vi "Test Comm.vi"() -> ()   [LabVIEW 2021]
uses:
  CIFChannels/Typedef/Direction.ctl
  ChannelCommon/typedef/FIFO Config.ctl
  ChannelCommon/typedef/Datatype Waveform.ctl
  ChannelCommon/typedef/TimeStamps.ctl
  CIF_NIChn_FIFO_DAQ.lvclass
  <vilib>/CIF Foundation/CIF Utilities/DataTypes/Flatten U64.vi
  ChannelCommon/ChannelCommon.lvlib
  CIFChannels/CIFChannels.lvclass
panel:
  out "status":string
  out "pass":bool
  out "error out":errorcluster
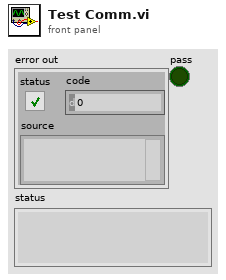
[diagram p1: front panel]
types:
  T1 = typedef "CIFChannels.lvclass/Direction.ctl" = enum16{"Publisher", "Subscriber"}
  T2 = typedef "ChannelCommon.lvlib/TimeStamps.ctl" = cluster{"ClockID":u8, "T0":i64, "T_Out":i64}
  T3 = typedef "ChannelCommon.lvlib/FIFO Config.ctl" = cluster{"Max Bytes/Msg":u64, "Max Msg/FIFO":u64, "Flags":u64}
  T4 = typedef "ChannelCommon.lvlib/Datatype Waveform.ctl" = cluster{"measurement":dbl[], "dT":dbl, "Timestamp":i64, "Read Lock":bool}
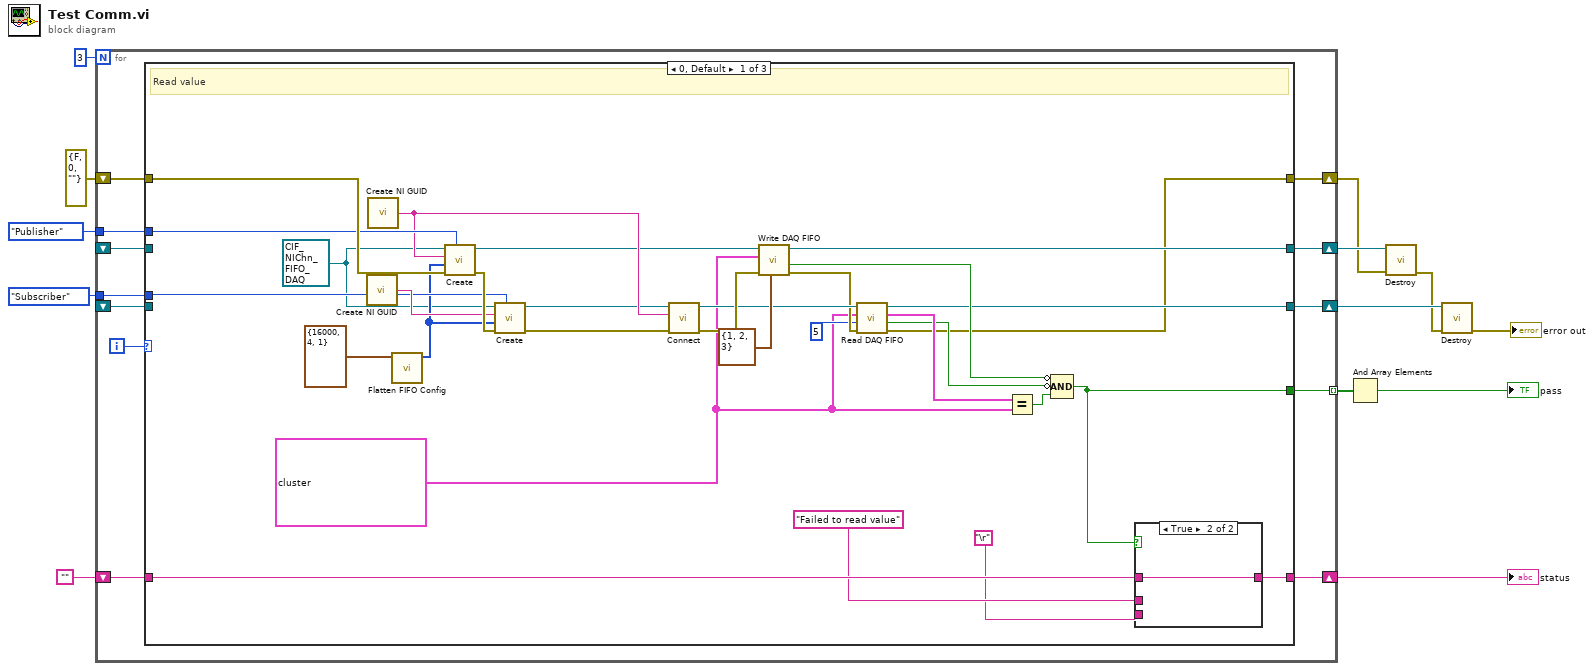
[diagram p0: block diagram]
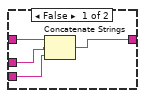
[diagram p2: hidden frame]
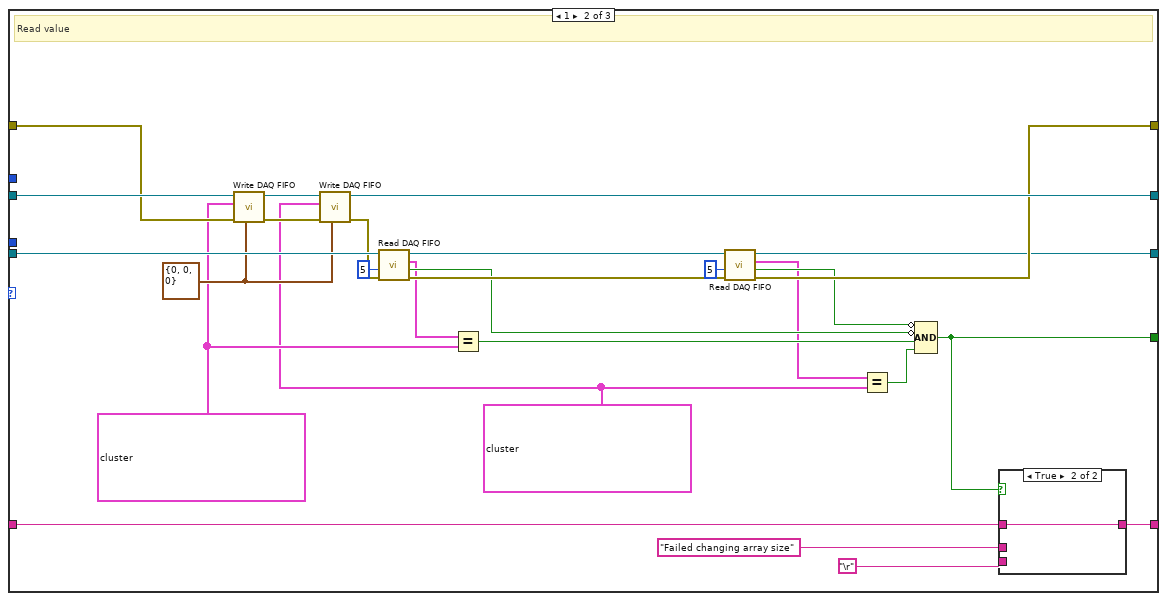
[diagram p3: hidden frame]
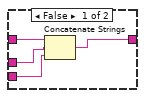
[diagram p4: hidden frame]
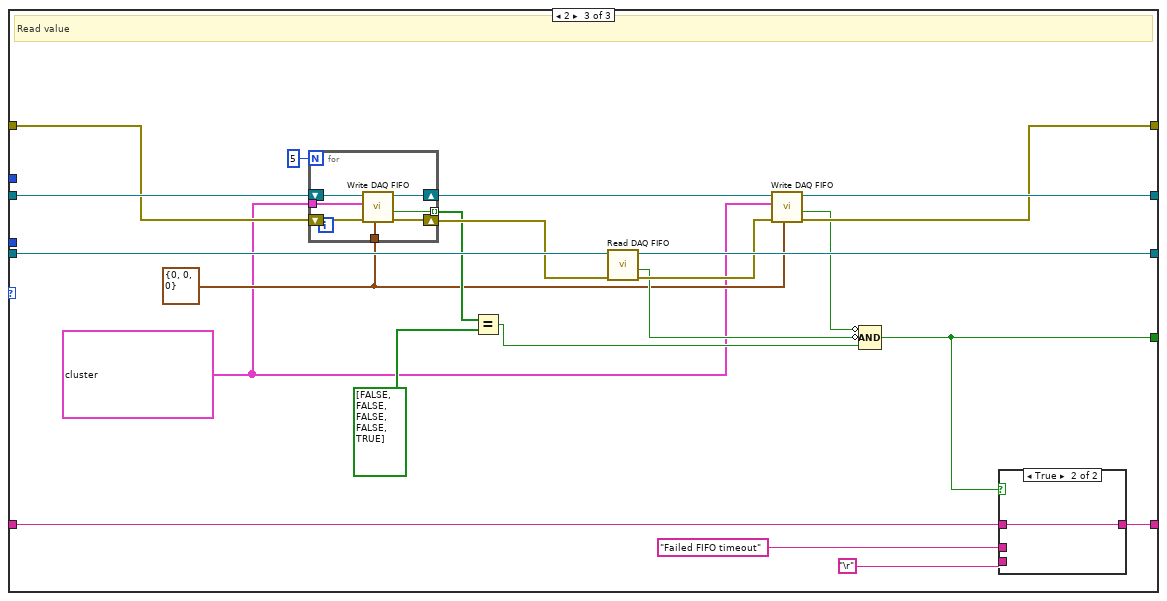
[diagram p5: hidden frame]
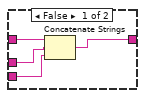
[diagram p6: hidden frame]
diagram:
  n1 = for {
    N: 3 -> [_]
    tunnel: [w25] -> w13 mode=indexing
    shift-right: [w14] -> w3
    shift-left: errorcluster {"status"=FALSE, "code"=0, "source"=""} ("error out") -> [w24]
    shift-right: [w21] -> w9
    shift-left: "" -> [w22]
    tunnel: Direction."Subscriber" ("Direction") -> [w20]
    tunnel: Direction."Publisher" ("Direction") -> [w19]
    shift-right: [w18] -> w5
    shift-left: _ -> [w16]
    shift-right: [w17] -> w4
    shift-left: _ -> [w15]
    i -> [w23]
    n2 = case shown="0, Default" w23 {
      tunnel: [w50 w83 w95] -> w25
      tunnel: w24 -> [w48 w79 w109]
      tunnel: [w28 w72 w101] -> w14
      tunnel: w22 -> [w55 w87 w114]
      tunnel: [w54 w86 w113] -> w21
      tunnel: w20 -> [w46 _ _]
      tunnel: w19 -> [w45 _ _]
      tunnel: [w30 w69 w106] -> w18
      tunnel: [w36 w76 w104] -> w17
      tunnel: w15 -> [_ w80 w110]
      tunnel: w16 -> [_ w75 w107]
      frame 0, Default {
        w26 = refnum<class "CIF_NIChn_FIFO_DAQ.lvclass"> refnum ("CIF_NIChn_FIFO_DAQ.lvclass")
        w27 = T4[] [{"measurement"=array[986 elements], "dT"=43.0, "Timestamp"=2, "Read Lock"=FALSE}, {"measurement"=array[1001 elements], "dT"=34.0, "Timestamp"=1, "Read Lock"=FALSE}] ("DAQ In")
        # "Read value"
        n3 = call <vilib>:"Create NI GUID.vi"() -> ("NI GUID"=w47:string)
        n4 = call <vilib>:"Create NI GUID.vi"() -> ("NI GUID"=w43:string)
        n5 = call "Flatten FIFO Config.vi"("FIFO Config in"=T3 {"Max Bytes/Msg"=16000, "Max Msg/FIFO"=4, "Flags"=1}) -> ("Flattened FIFO Config"=w40:u8[])  [unwired: 10 in]
        n6 = call-dynamic "Create.vi"("Direction"=w45, "error in (no error)"=w48, "Custom Config Data"=w40, "Name"=w43, "CIFFIFO in"=w26) -> ("error out"=w49:errorcluster, "CIFFIFO out"=w39:refnum<class "CIF_NIChn_FIFO_DAQ.lvclass">)  [unwired: 5 in]
        n7 = call-dynamic "Create.vi"("Direction"=w46, "error in (no error)"=w49, "Custom Config Data"=w40, "Name"=w47, "CIFFIFO in"=w26) -> ("error out"=w42:errorcluster, "CIFFIFO out"=w41:refnum<class "CIF_NIChn_FIFO_DAQ.lvclass">)  [unwired: 5 in]
        n8 = call-dynamic "Connect.vi"("error in (no error)"=w42, "Connection Name"=w43, "CIFTag in"=w41) -> ("error out"=w38:errorcluster, "CIFTag out"=w34:refnum<class "CIF_NIChn_FIFO_DAQ.lvclass">)  [unwired: 7 in]
        n9 = call-dynamic "Write DAQ FIFO.vi"("FIFO Timestamps"=T2 {"ClockID"=1, "T0"=2, "T_Out"=3}, "error in (no error)"=w38, "Data In"=w27, "CIF_NIChn_FIFO_DAQ in"=w39) -> ("error out"=w33:errorcluster, "timed out?"=w35:bool, "CIF_NIChn_FIFO_DAQ out"=w36:refnum<class "CIF_NIChn_FIFO_DAQ.lvclass">)  [unwired: 4 in, 1 out]
        n10 = call-dynamic "Read DAQ FIFO.vi"("error in (no error)"=w33, "Timeout (ms)"=5, "Data In"=w27, "CIF_NIChn_FIFO_DAQ in"=w34) -> ("error out"=w28:errorcluster, "timed out?"=w29:bool, "Data Out"=w31:T4[], "CIF_NIChn_FIFO_DAQ out"=w30:refnum<class "CIF_NIChn_FIFO_DAQ.lvclass">)  [unwired: 3 in, 1 out]
        n11 = Equal?(x=w31, y=w27) -> (x = y?=w51:bool)
        n12 = Compound Arithmetic op=AND(invert w35, invert w29, w51) -> (w50:bool)
        n13 = case shown="True" w50 {
          tunnel: w55 -> [w59 w60]
          tunnel: [w56 w60] -> w54
          tunnel: "Failed to read value" -> [w58 _]
          tunnel: "\r" -> [w57 _]
          frame False {
            n14 = Concatenate Strings(w59, w58, w57) -> (w56:string)
          }
          frame True {
          }
        }
      }
      frame 1 {
        w61 = T4[] [{"measurement"=array[986 elements], "dT"=213.0, "Timestamp"=2, "Read Lock"=FALSE}, {"measurement"=array[1001 elements], "dT"=32.0, "Timestamp"=1, "Read Lock"=FALSE}, {"measurement"=array[988 elements], "dT"=123.0, "Timestamp"=4, "Read Lock"=FALSE}] ("DAQ In")
        w62 = T4[] [{"measurement"=array[986 elements], "dT"=1.0, "Timestamp"=2, "Read Lock"=FALSE}, {"measurement"=array[1001 elements], "dT"=83.0, "Timestamp"=1, "Read Lock"=FALSE}, {"measurement"=array[988 elements], "dT"=78.0, "Timestamp"=4, "Read Lock"=FALSE}] ("DAQ In")
        w63 = T2 {"ClockID"=0, "T0"=0, "T_Out"=0} ("FIFO Timestamps")
        # "Read value"
        n15 = call-dynamic "Write DAQ FIFO.vi"("FIFO Timestamps"=w63, "error in (no error)"=w79, "Data In"=w62, "CIF_NIChn_FIFO_DAQ in"=w80) -> ("error out"=w77:errorcluster, "CIF_NIChn_FIFO_DAQ out"=w78:refnum<class "CIF_NIChn_FIFO_DAQ.lvclass">)  [unwired: 4 in, 2 out]
        n16 = call-dynamic "Write DAQ FIFO.vi"("FIFO Timestamps"=w63, "error in (no error)"=w77, "Data In"=w61, "CIF_NIChn_FIFO_DAQ in"=w78) -> ("error out"=w73:errorcluster, "CIF_NIChn_FIFO_DAQ out"=w76:refnum<class "CIF_NIChn_FIFO_DAQ.lvclass">)  [unwired: 4 in, 2 out]
        n17 = call-dynamic "Read DAQ FIFO.vi"("error in (no error)"=w73, "Timeout (ms)"=5, "CIF_NIChn_FIFO_DAQ in"=w75) -> ("error out"=w71:errorcluster, "timed out?"=w67:bool, "Data Out"=w64:T4[], "CIF_NIChn_FIFO_DAQ out"=w68:refnum<class "CIF_NIChn_FIFO_DAQ.lvclass">)  [unwired: 4 in, 1 out]
        n18 = Equal?(x=w64, y=w62) -> (x = y?=w81:bool)
        n19 = call-dynamic "Read DAQ FIFO.vi"("error in (no error)"=w71, "Timeout (ms)"=5, "CIF_NIChn_FIFO_DAQ in"=w68) -> ("error out"=w72:errorcluster, "timed out?"=w66:bool, "Data Out"=w65:T4[], "CIF_NIChn_FIFO_DAQ out"=w69:refnum<class "CIF_NIChn_FIFO_DAQ.lvclass">)  [unwired: 4 in, 1 out]
        n20 = Equal?(x=w65, y=w61) -> (x = y?=w82:bool)
        n21 = Compound Arithmetic op=AND(invert w66, invert w67, w81, w82) -> (w83:bool)
        n22 = case shown="True" w83 {
          tunnel: w87 -> [w91 w92]
          tunnel: [w88 w92] -> w86
          tunnel: "Failed changing array size" -> [w90 _]
          tunnel: "\r" -> [w89 _]
          frame False {
            n23 = Concatenate Strings(w91, w90, w89) -> (w88:string)
          }
          frame True {
          }
        }
      }
      frame 2 {
        w93 = T4[] [{"measurement"=array[986 elements], "dT"=43.0, "Timestamp"=2, "Read Lock"=FALSE}, {"measurement"=array[1001 elements], "dT"=34.0, "Timestamp"=1, "Read Lock"=FALSE}] ("DAQ In")
        w94 = T2 {"ClockID"=0, "T0"=0, "T_Out"=0} ("FIFO Timestamps")
        # "Read value"
        n24 = for {
          N: 5 -> [_]
          tunnel: w93 -> [w119]
          tunnel: w94 -> [w118]
          shift-right: [w117] -> w105
          shift-left: w110 -> [w121]
          tunnel: [w116] -> w100 mode=indexing
          shift-right: [w115] -> w103
          shift-left: w109 -> [w120]
          n25 = call-dynamic "Write DAQ FIFO.vi"("FIFO Timestamps"=w118, "error in (no error)"=w120, "Data In"=w119, "CIF_NIChn_FIFO_DAQ in"=w121) -> ("error out"=w115:errorcluster, "timed out?"=w116:bool, "CIF_NIChn_FIFO_DAQ out"=w117:refnum<class "CIF_NIChn_FIFO_DAQ.lvclass">)  [unwired: 4 in, 1 out]
        }
        n26 = Equal?(x=w100, y=bool[] [FALSE, FALSE, FALSE, FALSE, TRUE]) -> (x = y?=w96:bool)
        n27 = call-dynamic "Read DAQ FIFO.vi"("error in (no error)"=w103, "CIF_NIChn_FIFO_DAQ in"=w107) -> ("error out"=w102:errorcluster, "timed out?"=w98:bool, "CIF_NIChn_FIFO_DAQ out"=w106:refnum<class "CIF_NIChn_FIFO_DAQ.lvclass">)  [unwired: 5 in, 2 out]
        n28 = call-dynamic "Write DAQ FIFO.vi"("FIFO Timestamps"=w94, "error in (no error)"=w102, "Data In"=w93, "CIF_NIChn_FIFO_DAQ in"=w105) -> ("error out"=w101:errorcluster, "timed out?"=w97:bool, "CIF_NIChn_FIFO_DAQ out"=w104:refnum<class "CIF_NIChn_FIFO_DAQ.lvclass">)  [unwired: 4 in, 1 out]
        n29 = Compound Arithmetic op=AND(invert w97, invert w98, w96) -> (w95:bool)
        n30 = case shown="True" w95 {
          tunnel: w114 -> [w125 w126]
          tunnel: [w122 w126] -> w113
          tunnel: "Failed FIFO timeout" -> [w124 _]
          tunnel: "\r" -> [w123 _]
          frame False {
            n31 = Concatenate Strings(w125, w124, w123) -> (w122:string)
          }
          frame True {
          }
        }
      }
    }
  }
  "status" <- w9
  n32 = And Array Elements(Boolean array=w13) -> (logical AND=→"pass":bool)
  n33 = call-dynamic "Destroy.vi"("error in (no error)"=w3, "CIFFIFO in"=w4) -> ("error out"=w2:errorcluster)  [unwired: 8 in, 1 out]
  n34 = call-dynamic "Destroy.vi"("error in (no error)"=w2, "CIFFIFO in"=w5) -> ("error out"=→"error out":errorcluster)  [unwired: 8 in, 1 out]
